vi "ejemplo_mouse.vi"   [LabVIEW 2013]
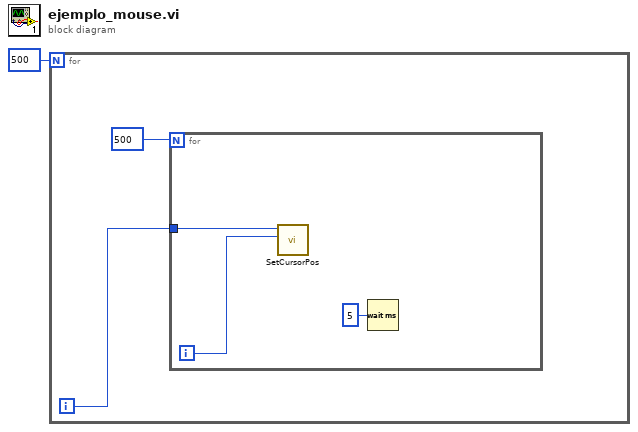
[diagram p0: block diagram]
diagram:
  n1 = for {
    N: 500 -> [_]
    i -> [w2]
    n2 = for {
      N: 500 -> [_]
      tunnel: w2 -> [w6]
      i -> [w5]
      n3 = call "SetCursorPos.vi"("dy"=w5, "dx"=w6) -> ()  [unwired: 10 in]
      n4 = Wait (ms)(milliseconds to wait=u32 5) -> ()  [unwired: 1 out]
    }
  }
